vi "CAMERA LIVE FEED FGV.vi"(7 "Enum - Menu":T1, 8 "error in (no error)":errorcluster, 9 "Image Path":string, 10 "CAMERA MODE":u8=48 format="%.0x", 11 "CAMERA PORT":u8=48) -> (0 "error out":errorcluster, 2 "data out":string)   [LabVIEW 2025]
uses:
  CAMERA LIVE FEED ENUM.ctl
  <vilib>/Utility/error.llb/Trim Whitespace One-Sided.vi
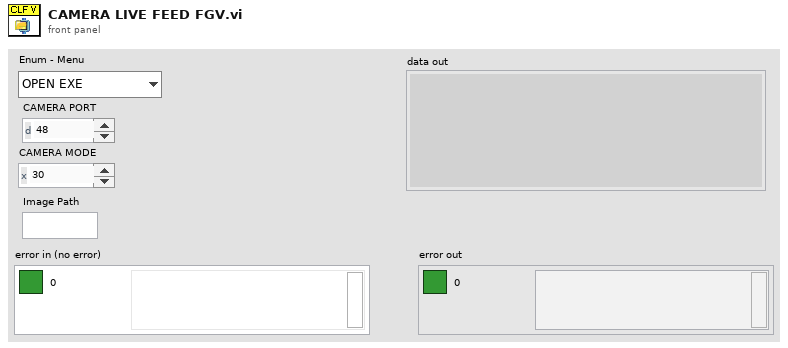
[diagram p1: front panel]
types:
  T1 = typedef "CAMERA LIVE FEED ENUM.ctl" = enum16{"OPEN EXE", "INIT", "READ", "CAMERA CONNECT", "CAMERA START", "CAMERA STOP", "CAMERA GRAY", "CAMERA RGB", "CAMERA MINIMIZE", "CAMERA CLOSE", "CAMERA MODE LIST", "CAMERA MODE SET", "CAMERA RESTORE", "CAMERA SAVE", "CLOSE"}
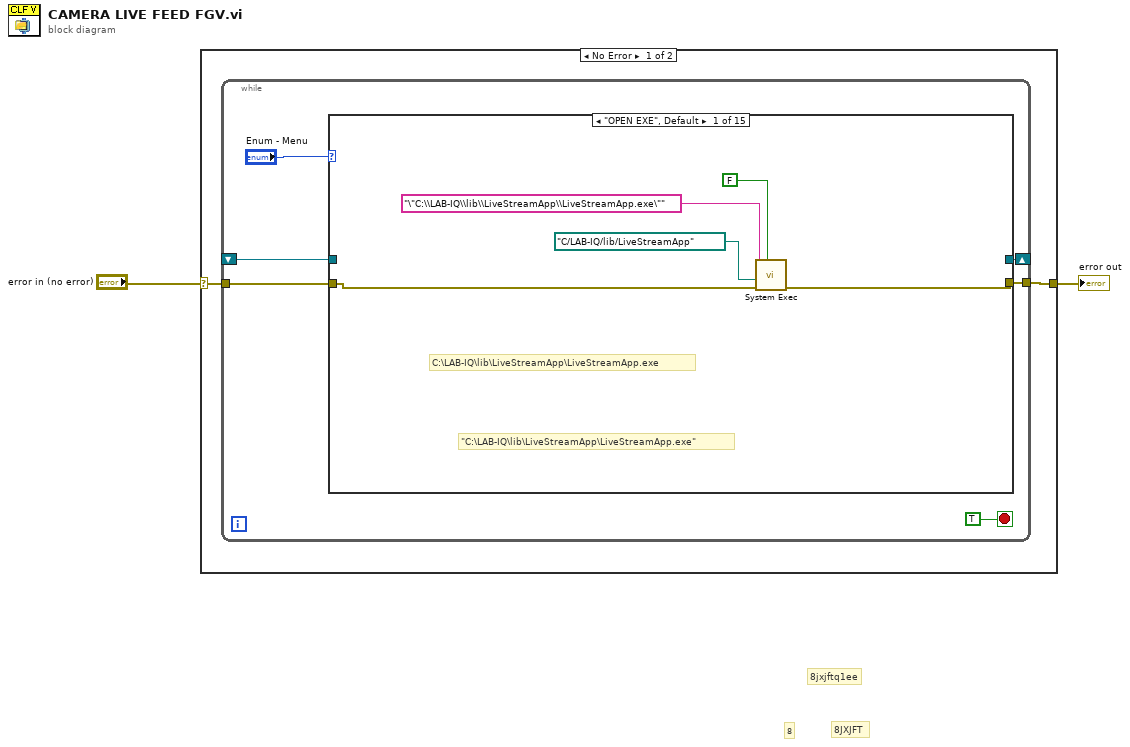
[diagram p0: block diagram]
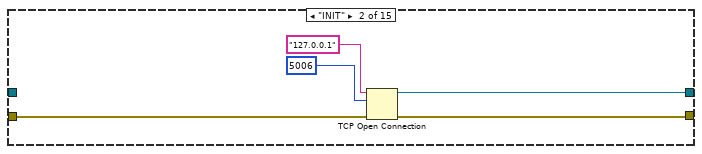
[diagram p2: hidden frame]
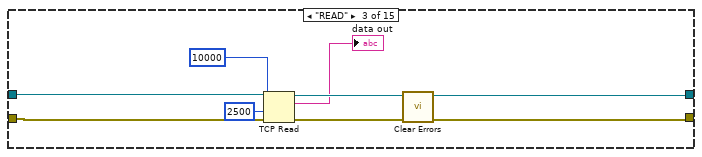
[diagram p3: hidden frame]
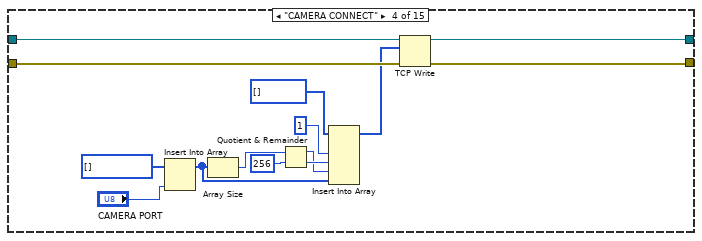
[diagram p4: hidden frame]
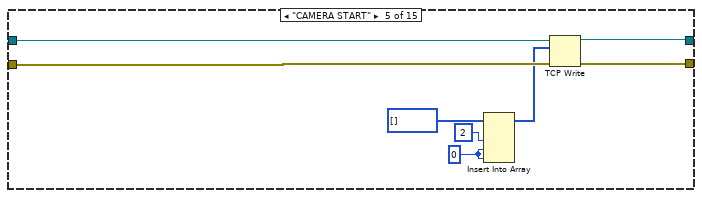
[diagram p5: hidden frame]
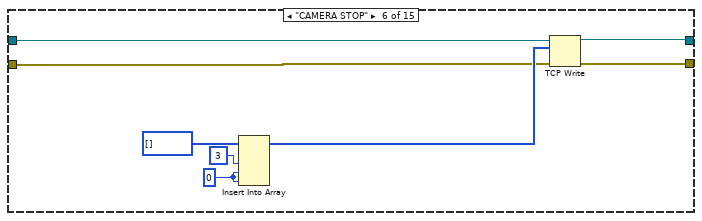
[diagram p6: hidden frame]
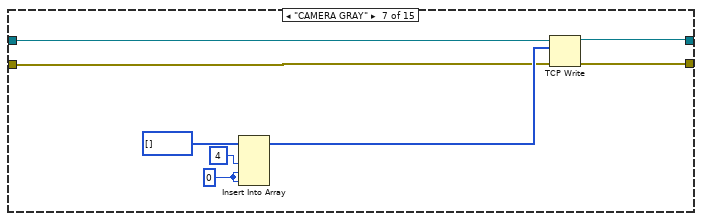
[diagram p7: hidden frame]
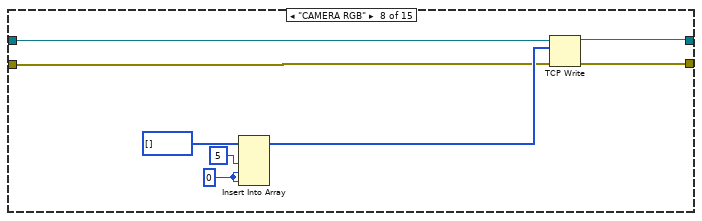
[diagram p8: hidden frame]
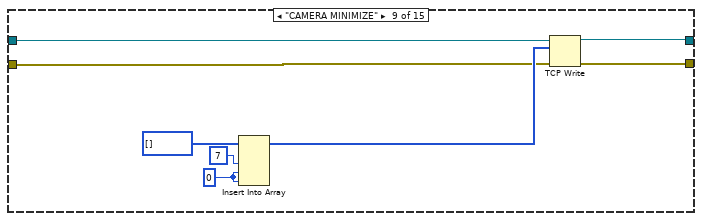
[diagram p9: hidden frame]
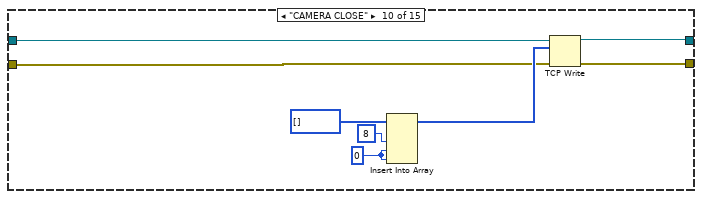
[diagram p10: hidden frame]
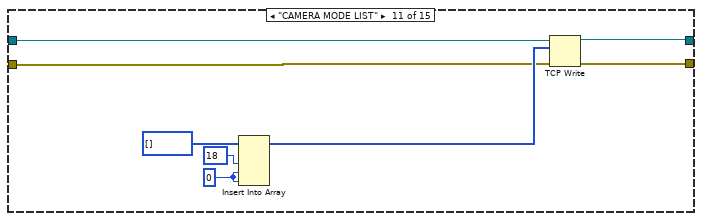
[diagram p11: hidden frame]
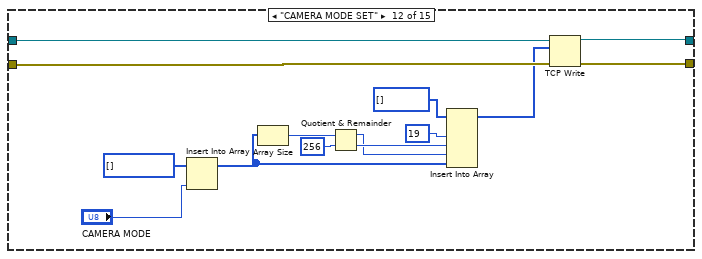
[diagram p12: hidden frame]
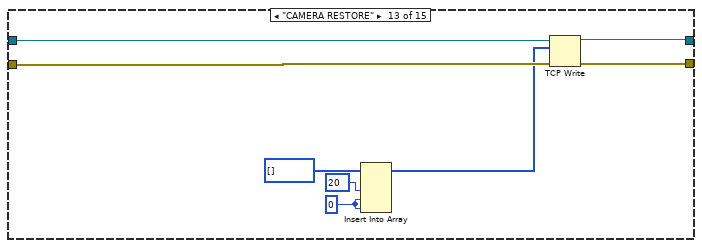
[diagram p13: hidden frame]
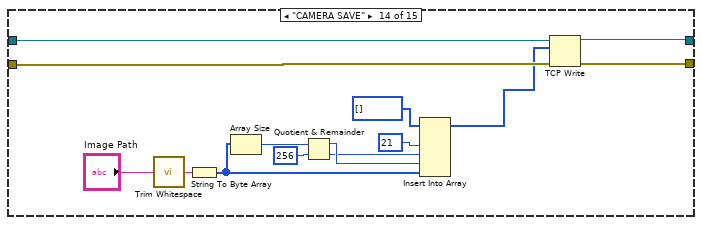
[diagram p14: hidden frame]
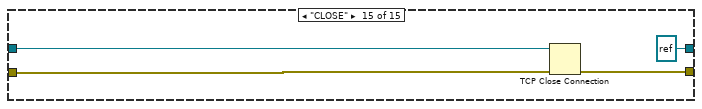
[diagram p15: hidden frame]
diagram:
  # "8JXJFT"
  # "8"
  # "8jxjftq1ee"
  n1 = case shown="No Error" "error in (no error)" {
    selector: "error in (no error)" -> [w4 _]
    tunnel: [w3 _] -> w1
    frame No Error {
      n2 = while {
        tunnel: w4 -> [w8]
        tunnel: [w7] -> w3
        shift-right: [w6] -> _
        shift-left: _ -> [w5]
        stop <- TRUE stop-if-true
        n3 = case shown="\"OPEN EXE\", Default" "Enum - Menu" {
          tunnel: w8 -> [w15 w18 w28 w30 w46 w53 w61 w69 w77 w85 w93 w111 w119 w133 w137]
          tunnel: [w14 w17 w21 w33 w47 w54 w62 w70 w78 w86 w94 w112 w120 w134 w138] -> w7
          tunnel: [_ w16 w23 w32 w44 w51 w59 w67 w75 w83 w91 w109 w117 w131 refnum<k5> refnum ("connection ID")] -> w6
          tunnel: w5 -> [_ _ w26 w31 w45 w52 w60 w68 w76 w84 w92 w110 w118 w132 w136]
          frame "OPEN EXE", Default {
            # "\"C:\\LAB-IQ\\lib\\LiveStreamApp\\LiveStreamApp.exe\""
            # "C:\\LAB-IQ\\lib\\LiveStreamApp\\LiveStreamApp.exe"
            n4 = call <vilib>:"System Exec.vi"("wait until completion? (T)"=FALSE, "error in (no error)"=w15, "working directory"=path "C:/LAB-IQ/lib/LiveStreamApp", "command line"="\"C:\\LAB-IQ\\lib\\LiveStreamApp\\LiveStreamApp.exe\"") -> ("error out"=w14:errorcluster)  [unwired: 4 in, 3 out]
          }
          frame "INIT" {
            n5 = TCP Open Connection(address="127.0.0.1", remote port or service name=u16 5006, error in (no error)=w18) -> (connection ID=w16:refnum<k5>, error out=w17:errorcluster)  [unwired: 2 in]
          }
          frame "READ" {
            n6 = TCP Read(connection ID=w26, bytes to read=10000, error in (no error)=w28, 9:2500 ("timeout ms (25000)")) -> (connection ID out=w23:refnum<k5>, data out=→"data out":string, error out=w27:errorcluster)  [unwired: 1 in]
            n7 = call <vilib>:"Clear Errors.vi"("error in (no error)"=w27) -> ("error out"=w21:errorcluster)  [unwired: 5 in, 1 out]
          }
          frame "CAMERA CONNECT" {
            n8 = Insert Into Array(array=u8[] [] ("unsigned byte array"), new element="CAMERA PORT") -> (w35:u8[])  [unwired: 1 in]
            n9 = Array Size(array=w35) -> (size(s)=w38:i32)
            n10 = Quotient & Remainder(x=w38, y=256) -> (x-y*floor(x/y)=w39:i32, floor(x/y)=w40:i32)
            n11 = Insert Into Array(array=u8[] [] ("unsigned byte array"), new element #1=1, new element #2=w40, new element #3=w39, new element #4=w35) -> (w29:u8[])  [unwired: 1 in]
            n12 = TCP Write(connection ID=w31, data in=w29, error in (no error)=w30) -> (connection ID out=w32:refnum<k5>, error out=w33:errorcluster)  [unwired: 1 in, 1 out]
          }
          frame "CAMERA START" {
            w50 = 0
            n13 = Insert Into Array(array=u8[] [] ("unsigned byte array"), new element #1=u8 2 ("codes"), new element #2=w50, new element #3=w50) -> (w43:u8[])  [unwired: 1 in]
            n14 = TCP Write(connection ID=w45, data in=w43, error in (no error)=w46) -> (connection ID out=w44:refnum<k5>, error out=w47:errorcluster)  [unwired: 1 in, 1 out]
          }
          frame "CAMERA STOP" {
            w58 = 0
            n15 = Insert Into Array(array=u8[] [] ("unsigned byte array"), new element #1=u8 3 ("codes"), new element #2=w58, new element #3=w58) -> (w55:u8[])  [unwired: 1 in]
            n16 = TCP Write(connection ID=w52, data in=w55, error in (no error)=w53) -> (connection ID out=w51:refnum<k5>, error out=w54:errorcluster)  [unwired: 1 in, 1 out]
          }
          frame "CAMERA GRAY" {
            w66 = 0
            n17 = Insert Into Array(array=u8[] [] ("unsigned byte array"), new element #1=u8 4 ("codes"), new element #2=w66, new element #3=w66) -> (w63:u8[])  [unwired: 1 in]
            n18 = TCP Write(connection ID=w60, data in=w63, error in (no error)=w61) -> (connection ID out=w59:refnum<k5>, error out=w62:errorcluster)  [unwired: 1 in, 1 out]
          }
          frame "CAMERA RGB" {
            w74 = 0
            n19 = Insert Into Array(array=u8[] [] ("unsigned byte array"), new element #1=u8 5 ("codes"), new element #2=w74, new element #3=w74) -> (w71:u8[])  [unwired: 1 in]
            n20 = TCP Write(connection ID=w68, data in=w71, error in (no error)=w69) -> (connection ID out=w67:refnum<k5>, error out=w70:errorcluster)  [unwired: 1 in, 1 out]
          }
          frame "CAMERA MINIMIZE" {
            w82 = 0
            n21 = Insert Into Array(array=u8[] [] ("unsigned byte array"), new element #1=u8 7 ("codes"), new element #2=w82, new element #3=w82) -> (w79:u8[])  [unwired: 1 in]
            n22 = TCP Write(connection ID=w76, data in=w79, error in (no error)=w77) -> (connection ID out=w75:refnum<k5>, error out=w78:errorcluster)  [unwired: 1 in, 1 out]
          }
          frame "CAMERA CLOSE" {
            w90 = 0
            n23 = Insert Into Array(array=u8[] [] ("unsigned byte array"), new element #1=u8 8 ("codes"), new element #2=w90, new element #3=w90) -> (w87:u8[])  [unwired: 1 in]
            n24 = TCP Write(connection ID=w84, data in=w87, error in (no error)=w85) -> (connection ID out=w83:refnum<k5>, error out=w86:errorcluster)  [unwired: 1 in, 1 out]
          }
          frame "CAMERA MODE LIST" {
            w98 = 0
            n25 = Insert Into Array(array=u8[] [] ("unsigned byte array"), new element #1=u8 18 ("codes"), new element #2=w98, new element #3=w98) -> (w95:u8[])  [unwired: 1 in]
            n26 = TCP Write(connection ID=w92, data in=w95, error in (no error)=w93) -> (connection ID out=w91:refnum<k5>, error out=w94:errorcluster)  [unwired: 1 in, 1 out]
          }
          frame "CAMERA MODE SET" {
            n27 = Insert Into Array(array=u8[] [] ("unsigned byte array"), new element="CAMERA MODE") -> (w100:u8[])  [unwired: 1 in]
            n28 = Array Size(array=w100) -> (size(s)=w103:i32)
            n29 = Quotient & Remainder(x=w103, y=256) -> (x-y*floor(x/y)=w104:i32, floor(x/y)=w105:i32)
            n30 = Insert Into Array(array=u8[] [] ("unsigned byte array"), new element #1=19, new element #2=w105, new element #3=w104, new element #4=w100) -> (w102:u8[])  [unwired: 1 in]
            n31 = TCP Write(connection ID=w110, data in=w102, error in (no error)=w111) -> (connection ID out=w109:refnum<k5>, error out=w112:errorcluster)  [unwired: 1 in, 1 out]
          }
          frame "CAMERA RESTORE" {
            w116 = 0
            n32 = Insert Into Array(array=u8[] [] ("unsigned byte array"), new element #1=u8 20 ("codes"), new element #2=w116, new element #3=w116) -> (w113:u8[])  [unwired: 1 in]
            n33 = TCP Write(connection ID=w118, data in=w113, error in (no error)=w119) -> (connection ID out=w117:refnum<k5>, error out=w120:errorcluster)  [unwired: 1 in, 1 out]
          }
          frame "CAMERA SAVE" {
            n34 = call <vilib>:"Trim Whitespace.vi"("string"="Image Path") -> ("trimmed string"=w121:string)  [unwired: 1 in]
            n35 = String To Byte Array(string=w121) -> (unsigned byte array=w126:u8[])
            n36 = Array Size(array=w126) -> (size(s)=w128:i32)
            n37 = Quotient & Remainder(x=w128, y=256) -> (x-y*floor(x/y)=w125:i32, floor(x/y)=w124:i32)
            n38 = Insert Into Array(array=u8[] [] ("unsigned byte array"), new element #1=21, new element #2=w124, new element #3=w125, new element #4=w126) -> (w123:u8[])  [unwired: 1 in]
            n39 = TCP Write(connection ID=w132, data in=w123, error in (no error)=w133) -> (connection ID out=w131:refnum<k5>, error out=w134:errorcluster)  [unwired: 1 in, 1 out]
          }
          frame "CLOSE" {
            n40 = TCP Close Connection(connection ID=w136, error in (no error)=w137) -> (error out=w138:errorcluster)  [unwired: 1 in, 1 out]
          }
        }
      }
    }
    frame Error {
    }
  }
  "error out" <- w1
